vi "Laser_tcp_task.vi"(9 "bytes to read":i32=186, 10 "queue out":refnum<queue>, 11 "address":string) -> (3 "Data size":u32)   [LabVIEW 2023]
uses:
  TypeDefs/laser_cabinet_status.ctl
  Globals/Globals.vi
  Get_Laser_Cabinet_Status.vi
panel:
  in  "milliseconds to wait":u32=1000
  out "Status":T1(ring)
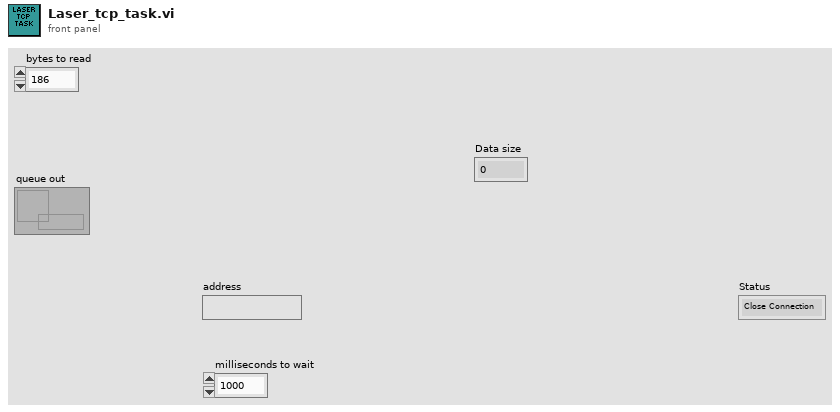
[diagram p1: front panel]
types:
  T1 = enum16{"Close Connection", "Connected", "Create Connection"}
  T2 = typedef "LaserTrain_config.ctl" = cluster{"Blower Configuration":T3, "Chiller Configuration":T4, "Pneumatics Configuration":T5, "UPS Configuration":T6, "Network":T7, "Laser Config":T8}
  T3 = typedef "Blower_config.ctl" = cluster{"Pressure min":dbl, "Pressure max":dbl, "Startup Timer":dbl, "Interval Timer":dbl}
  T4 = typedef "Chiller_config.ctl" = cluster{"Flow min (Low Temp Loop)":dbl, "Flow min (High Temp Loop)":dbl, "Temperature Setpoint min":dbl, "Temperature Setpoint max":dbl, "Temperature Offset":dbl, "Safety Temperature":dbl, "Dew Point Margin":dbl, "Dew Point Margin Extra":dbl, "Flow Minimum Timer":dbl}
  T5 = typedef "Pneumatics_config.ctl" = cluster{"Pressure Startup":dbl, "Pressure min":dbl, "Pressure max":dbl, "Fill Wet Tank Timer":dbl, "Fill Dry Tank Timer":dbl, "Fill Wet Tank Timer Retry":dbl, "Fill Dry Tank Timer Retry":dbl, "Blow Off Timer":dbl}
  T6 = typedef "Ups_config.ctl" = cluster{"Connection Time":dbl}
  T7 = typedef "Network_config.ctl" = cluster{"cRIO IP":string, "Laser N1 IP":string, "Laser N2 IP":string, "Laser S1 IP":string, "Laser S2 IP":string, "GPS Pi IP":string, "Camera N Pi IP":string, "Camera S Pi IP":string, "Chiller N IP":string, "Chiller S IP":string, "UPS IP":string}
  T8 = typedef "Laser_config.ctl" = cluster{"Power":sgl, "Min PRR":sgl, "Max PRR":sgl}
  T9 = typedef "GPS.ctl" = cluster{"Data received":bool, "All":bool, "Area":bool, "Crossing":bool, "Bridges":bool, "Switch":bool, "Speed Min Ok":bool, "Speed Max Ok":bool, "Track":bool, "Quality":dbl, "Dilution of precision":dbl, "N Satelites":dbl, "Speed":dbl, "Lon":dbl, "Lat":dbl, "Detectors":bool, "Lubricators Acurate":bool, "Lubricators Estimate":bool, "Acces Pads":bool, "Manual Points":bool}
  T10 = typedef "laser_cabinet_status.ctl" = cluster{"Version":u16, "Installed Status":u32, "Set Mode Index":u16, "Set Frequency (kHz)":sgl, "Average Power (W)":sgl, "Set Power (%)":sgl, "Main Status":u32, "Alarms":u32, "System Alarms":u32, "Extended Alarms":u32, "Warnings":u32, "Status":u32, "Extended Status":u32, "Reserved1":u16, "Measured Frequency (kHz)":sgl, "Pulse Duration (ns)":u32, "Measured Power (W)":sgl, "Pulse Energy (mJ)":sgl, "Peak Power (kW)":sgl, "Analog power control (mV)":sgl, "Back Reflection (mV)":sgl, "PS mean (C)":sgl, "PS max (C)":sgl, "PS min (C)":sgl, "Dew Point (C)":sgl, "Remote Controller Temperature (C)":sgl, "Isolator Temperature (C)":sgl, "MO mean (C)":sgl, "MO max (C)":sgl, "MO min (C)":sgl, "PA mean (C)":sgl, "PA max (C)":sgl, "PA min (C)":sgl, "BS mean (C)":sgl, "BS max (C)":sgl, "BS min (C)":sgl, "Humidity (%)":sgl}
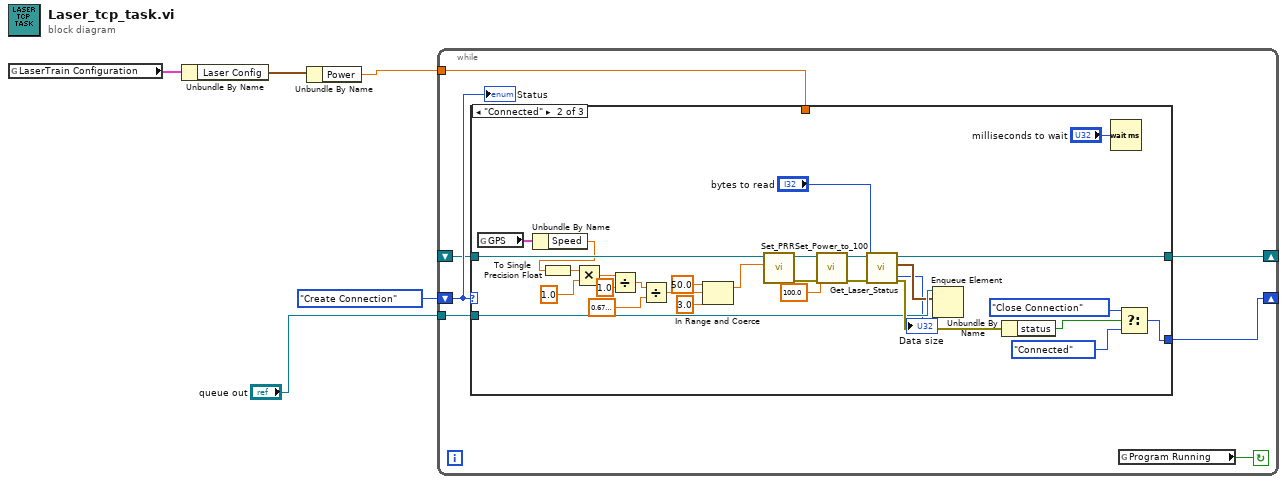
[diagram p0: block diagram]
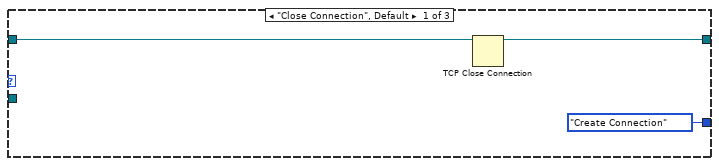
[diagram p2: hidden frame]
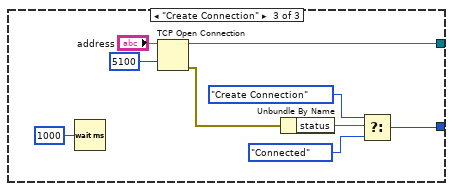
[diagram p3: hidden frame]
diagram:
  n1 = global read "Globals.vi" "LaserTrain Configuration"() -> (w3:T2)
  n2 = Unbundle By Name(w3) -> ("Laser Config"=w2:T8)
  n3 = Unbundle By Name(w2) -> ("Power"=w1:sgl)
  n4 = while {
    shift-right: [w9] -> _
    shift-left: T1."Create Connection" ("Enum") -> [w12]
    shift-right: [w11] -> _
    shift-left: _ -> [w10]
    tunnel: "queue out" -> [w8]
    tunnel: w1 -> [w6]
    stop <- w7 continue-if-true
    n5 = case shown="\"Connected\"" w12 {
      tunnel: [w14 w44 w52] -> w11
      tunnel: w10 -> [w15 w36 _]
      tunnel: [T1."Create Connection" ("Enum") w42 w49] -> w9
      tunnel: w8 -> [_ w37 _]
      tunnel: w6 -> [_ _ _]
      frame "Close Connection", Default {
        n6 = TCP Close Connection(connection ID=w15) -> (connection ID out=w14:refnum<k5>)  [unwired: 2 in, 1 out]
      }
      frame "Connected" {
        n7 = global read "Globals.vi" "GPS"() -> (w22:T9)
        n8 = Unbundle By Name(w22) -> ("Speed"=w28:dbl)
        n9 = To Single Precision Float(number=w28) -> (single precision float=w33:sgl)
        n10 = Multiply(x=w33, y=sgl 1.0) -> (x*y=w34:sgl)
        n11 = Divide(x=w34, y=sgl 1.0) -> (x/y=w35:sgl)
        n12 = Divide(x=w35, y=sgl 0.67) -> (x/y=w29:sgl)
        n13 = In Range and Coerce(upper limit=sgl 50.0, x=w29, lower limit=sgl 3.0) -> (coerced(x)=w21:sgl)  [unwired: 1 out]
        n14 = call "Set_PRR.vi"("PRR"=w21, "connection ID"=w36) -> ("error out"=w24:errorcluster, "connection ID out"=w27:refnum<k5>)  [unwired: 7 in, 1 out]
        n15 = call "Set_Power_to_100.vi"("error in (no error)"=w24, "Power (%)"=sgl 100.0, "connection ID"=w27) -> ("error out"=w25:errorcluster, "connection ID out"=w26:refnum<k5>)  [unwired: 5 in]
        n16 = call "Get_Laser_Status.vi"("error in (no error)"=w25, "bytes to read"="bytes to read", "connection ID"=w26) -> ("error out"=w43:errorcluster, "output cluster"=w23:T10, "connection ID out"=w44:refnum<k5>, "Data size"=→"Data size":u32)  [unwired: 4 in, 1 out]
        n17 = Enqueue Element(queue=w37, element=w23) -> ()  [unwired: 2 in, 3 out]
        n18 = Unbundle By Name(w43) -> ("status"=w41:bool)
        n19 = Wait (ms)(milliseconds to wait="milliseconds to wait") -> ()  [unwired: 1 out]
        n20 = Select(t=T1."Close Connection", s=w41, f=T1."Connected" ("Enum")) -> (s? t:f=w42:T1)
      }
      frame "Create Connection" {
        n21 = Wait (ms)(milliseconds to wait=u32 1000) -> ()  [unwired: 1 out]
        n22 = TCP Open Connection(address="address", remote port or service name=u16 5100) -> (connection ID=w52:refnum<k5>, error out=w51:errorcluster)  [unwired: 3 in]
        n23 = Unbundle By Name(w51) -> ("status"=w50:bool)
        n24 = Select(t=T1."Create Connection" ("Enum"), s=w50, f=T1."Connected" ("Enum")) -> (s? t:f=w49:T1)
      }
    }
    n25 = global read "Globals.vi" "Program Running"() -> (w7:bool)
    "Status" <- w12
  }
